vi "Go.vi"() -> ()   [LabVIEW 2011]
uses:
  <vilib>/Math Plots/2D Math Plots/2D Compass/2D Compass Datatype/Public/Plot Helper (Vector).vi
  <vilib>/Utility/file.llb/Read From Spreadsheet File (I64).vi
  <vilib>/Utility/file.llb/Write To Spreadsheet File (I64).vi
  <vilib>/robotics/Navigation/shared/WorldMap/OccupancyGridWorldMap/NI_Robotics_OccupancyGridWorldMap.lvclass
  <vilib>/robotics/Navigation/NI_Robotics_Navigation .lvlib
  <vilib>/robotics/Obstacle Avoidance/Simple Vector Field Histogram/NI_Robotics_Simple Vector Field Histogram.lvlib
  <vilib>/ptbypt/NI_PtbyPt.lvlib
  <vilib>/Math Plots/2D Math Plots/2D Compass/2D Compass Datatype/2D Compass Datatype.lvclass
panel:
  out "currentCoord":cluster{"x curr":i32, "y curr":i32}
  in  "uncertaintyList":u16(ring) caption="uncertainty" items=[" ", "Uncertainty", "Full"]
  in  "startCoord":cluster{"x start":i32, "y start":i32}
  in  "goalCoord":cluster{"x goal":i32, "y goal":i32}
  in  "Stop Button":bool
  in  "dimention":cluster{"x dim":dbl, "y dim":dbl}={"x dim"=100.0, "y dim"=100.0}
  in  "algoritms":u16(ring) items=["", "Dejkstra", "A*"]
  in  "Uncertain":u32(colorbox)=16448250
  in  "path":u32(colorbox) caption="Path"
  in  "goal":u32(colorbox)=16711744 caption="Goal"
  in  "start":u32(colorbox)=3381759 caption="Start"
  in  "invObs":u32(colorbox)=7171459 caption="Invisible"
  in  "visObs":u32(colorbox)=1985280 caption="Visible"
  in  "free":u32(colorbox)=13238105 caption="Free"
  out "enviroment":i32[][](graph)
  out "phArr":dbl[](array[numeric])
  out "magArr":dbl[](array[numeric])
  out "phase":dbl format="%0.2f"
  out "magnitude":dbl format="%0.2f"
  out "uncertainCode":i32
  out "pathCode":i32
  out "invObsCode":i32
  out "goalCode":i32
  out "startCode":i32
  out "visObsCode":i32
  out "freeCode":i32
  in  "?":T1(tab)
  in  "ModeOfGeneration":u16(ring) items=["Auto", "Hand", "Load"]
  in  "Listbox":i32(listbox)=1
  in  "Tree":string[](tree)
  in  "add":bool
  in  "del":bool
  in  "clear":bool
  in  "generation":bool
  in  "Density":i32=5
  in  "save":bool
  out "Scanning":bool=TRUE
  out "ActivePane":bool=TRUE
  in  "Numeric":dbl
  out "RM":bool
  out "LM":bool
  out "Sonar":bool
  out "Gauge":dbl(knob) scale=0.0..1.0
  out "?":dbl
  out "Slide":u8(slide) scale=0.0..100.0
  in  "Scanning Step":dbl=2.0
  out "2D Compass":cluster{dbl[], dbl[]}(graph)
  in  "stop":bool
  in  "Blank Button":bool
  out "path cost":dbl
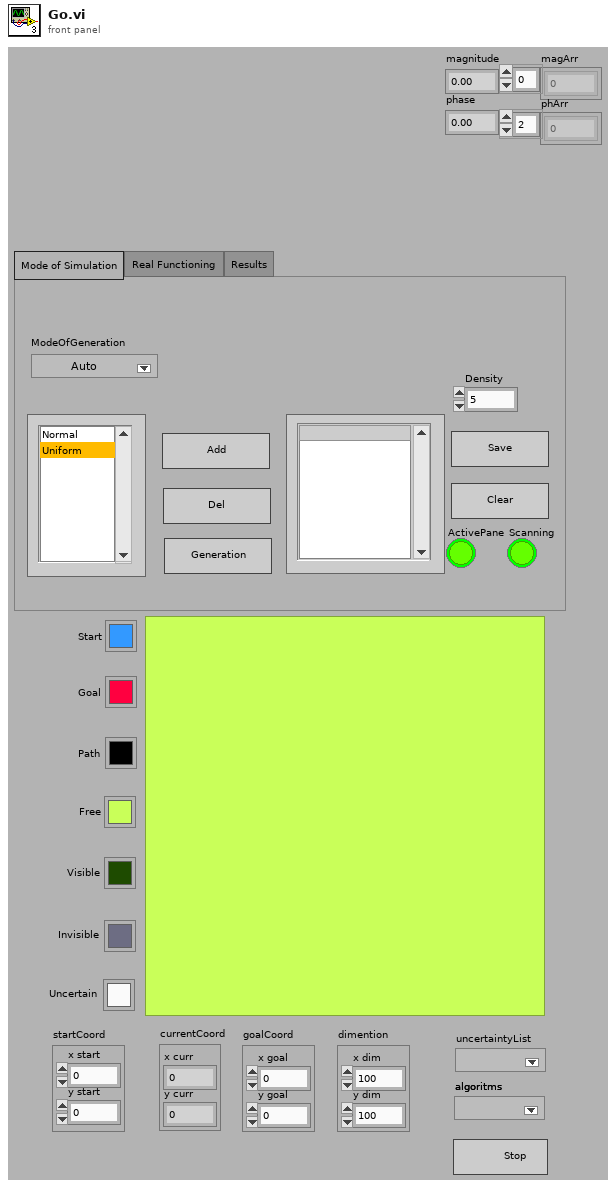
[diagram p1: front panel]
types:
  T1 = enum32{"Mode of Simulation", "Real Functioning ", "Results"}
  T2 = enum8{"Enabled", "Disabled", "Disabled and Grayed Out"}
  T3 = typedef "LVPoint32TypeDef.ctl" = cluster{"Horizontal":i32, "Vertical":i32}
  T4 = cluster{"min mag":dbl, "min phase":dbl, "max phase":dbl, "x relat":i32, "y relat":i32, "visible":bool, "full":bool, "detec":bool}[]
  T5 = typedef "NI_Robotics_Simple Vector Field Histogram.lvlib/Obstacle Description.ctl" = cluster{"angle to obstacle":dbl, "distance to obstacle":dbl}
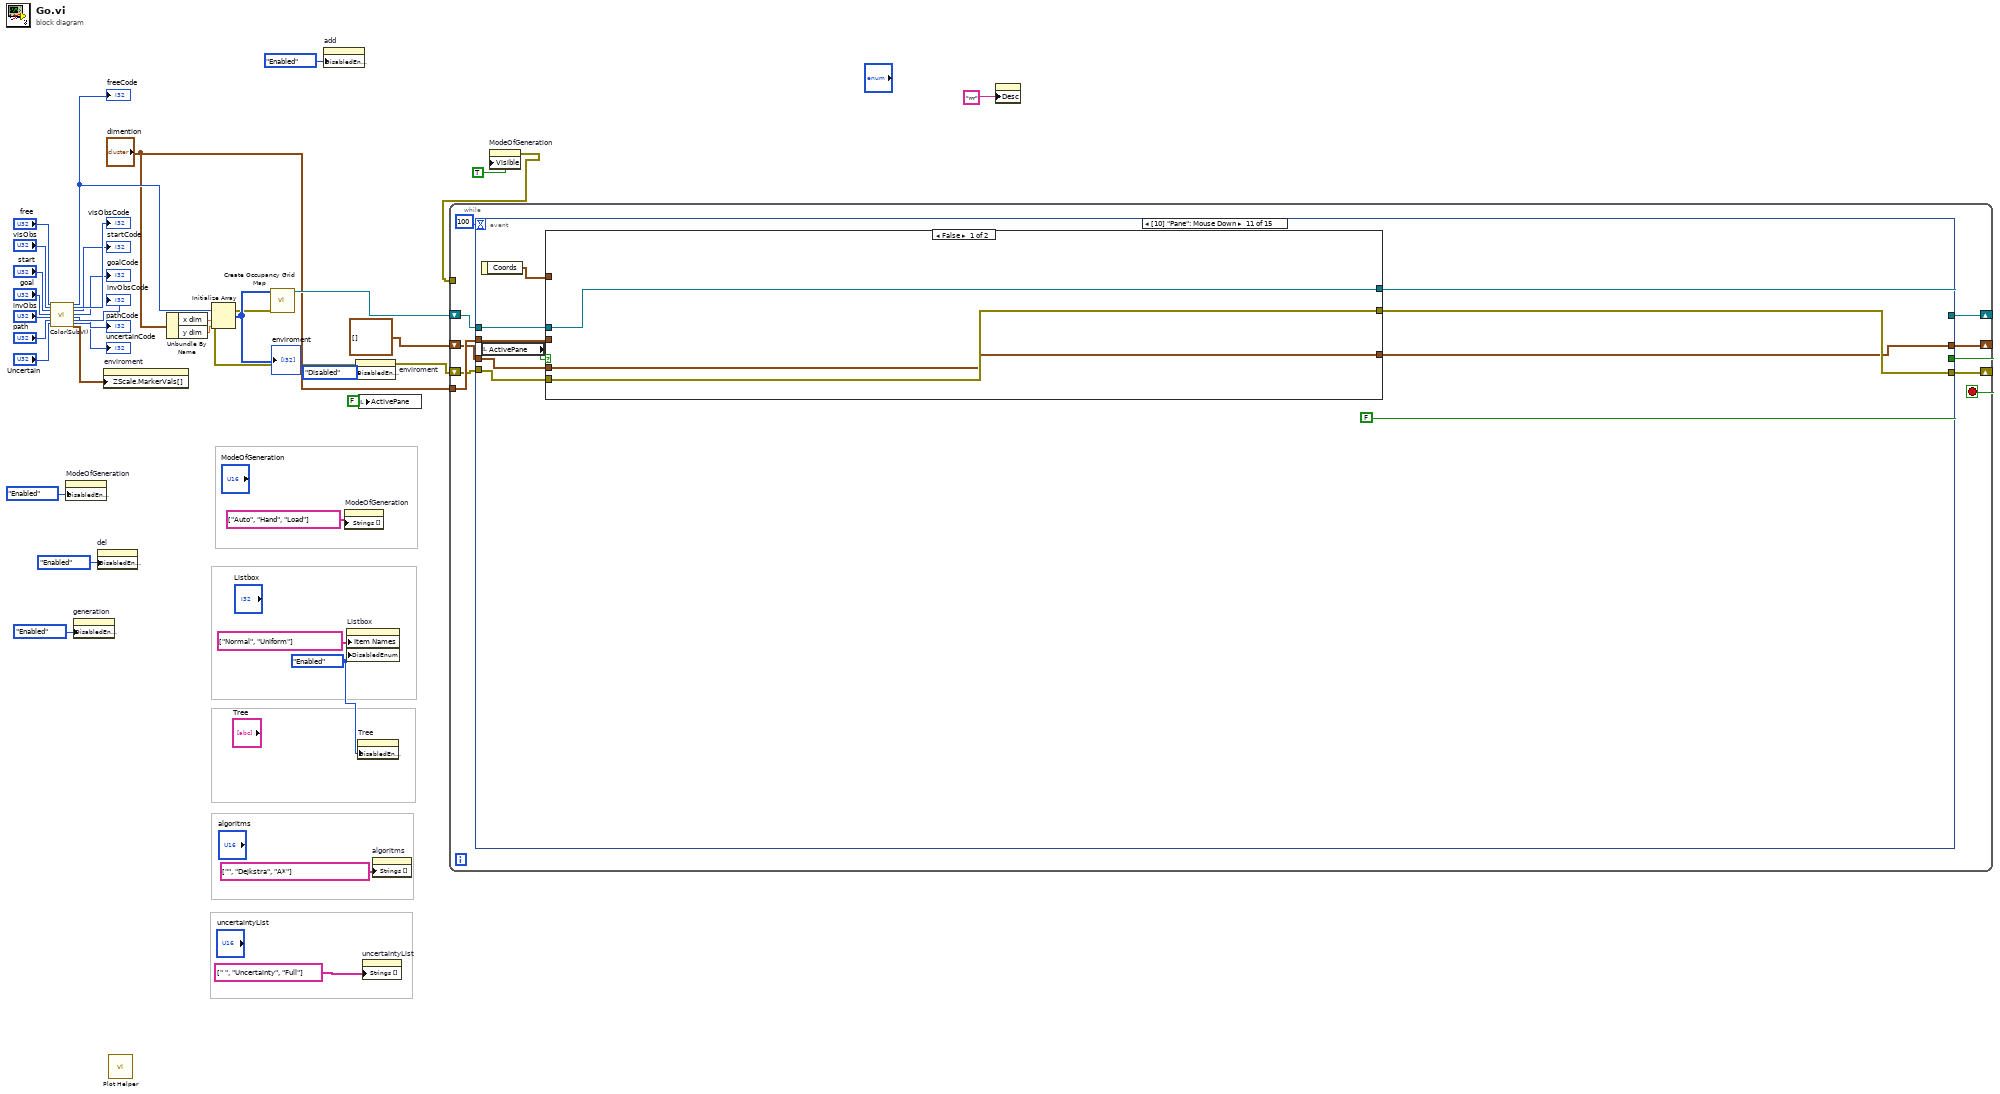
[diagram p0: block diagram]
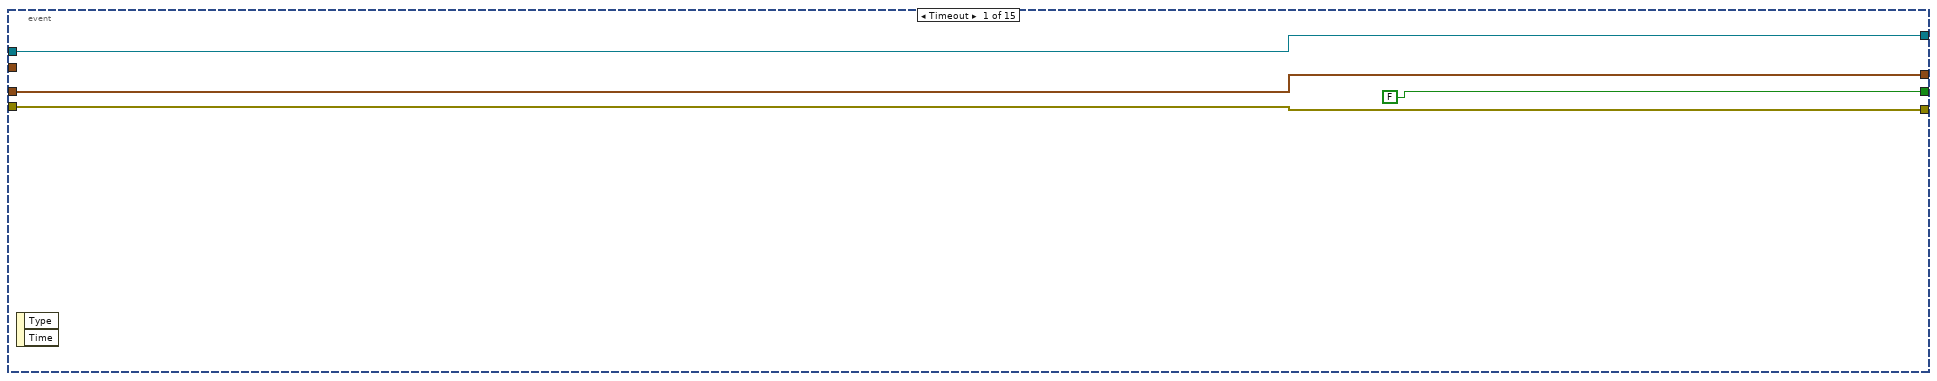
[diagram p2: hidden frame]
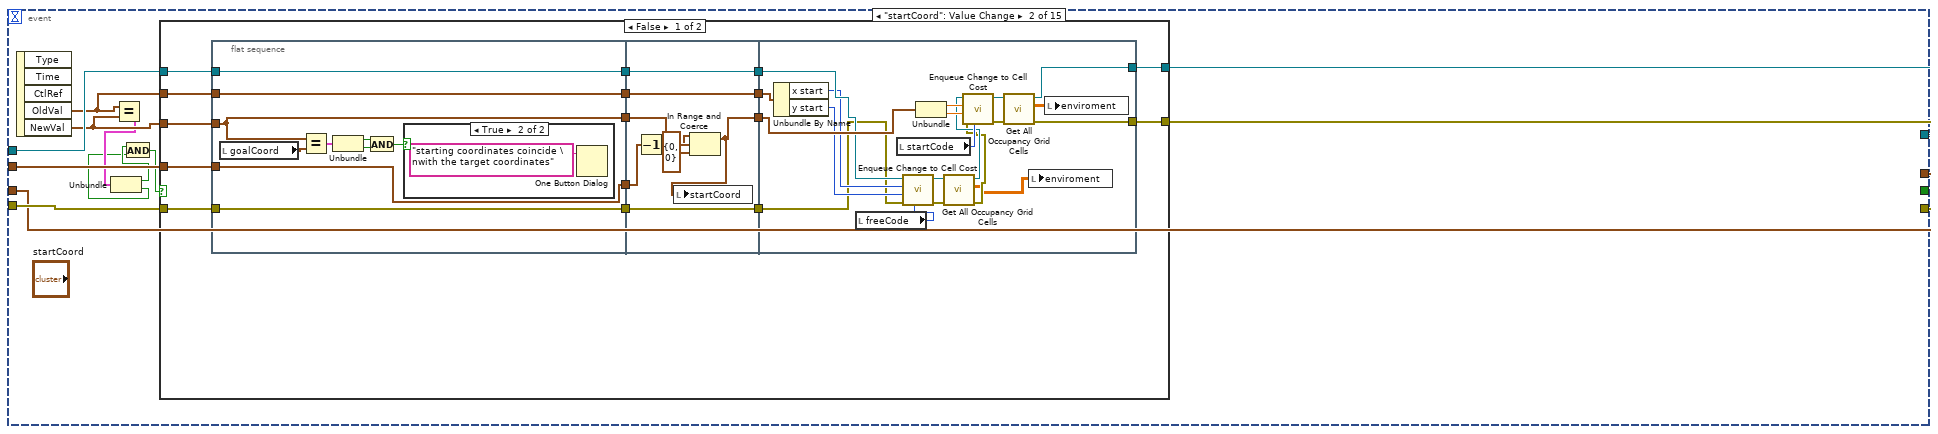
[diagram p3: hidden frame]
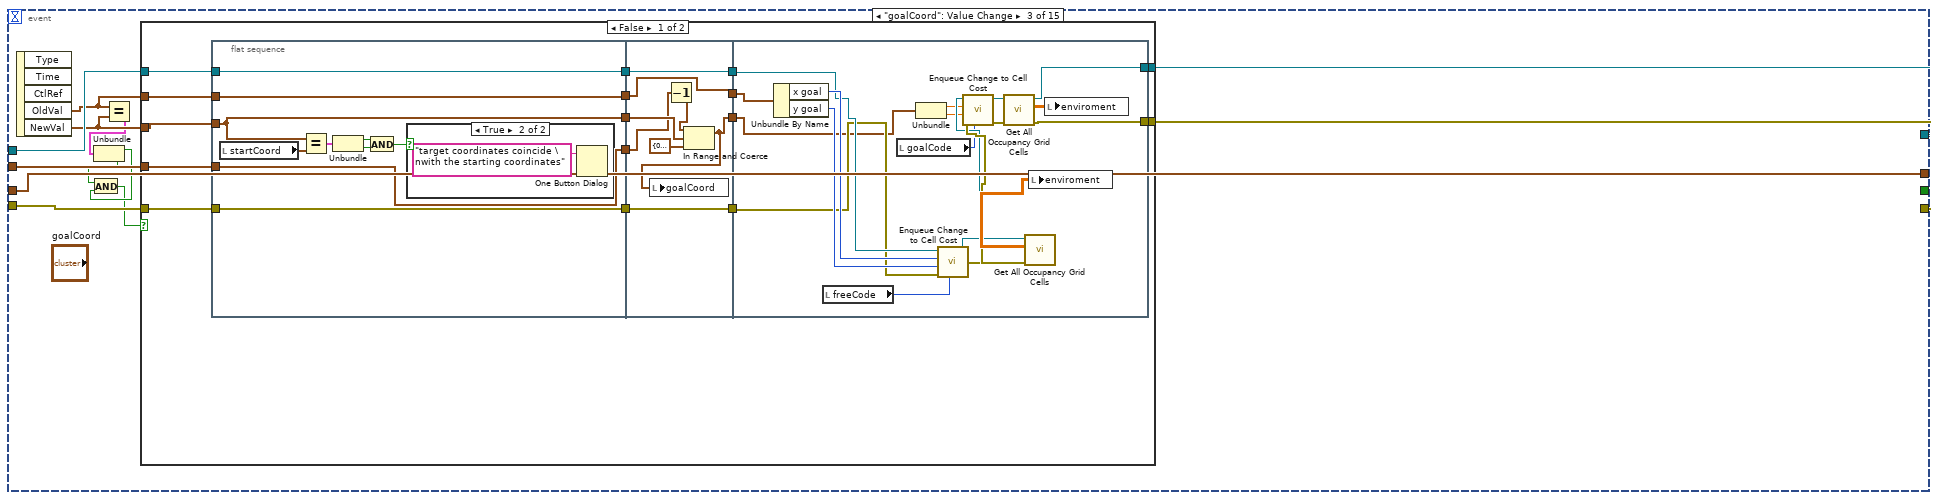
[diagram p6: hidden frame]
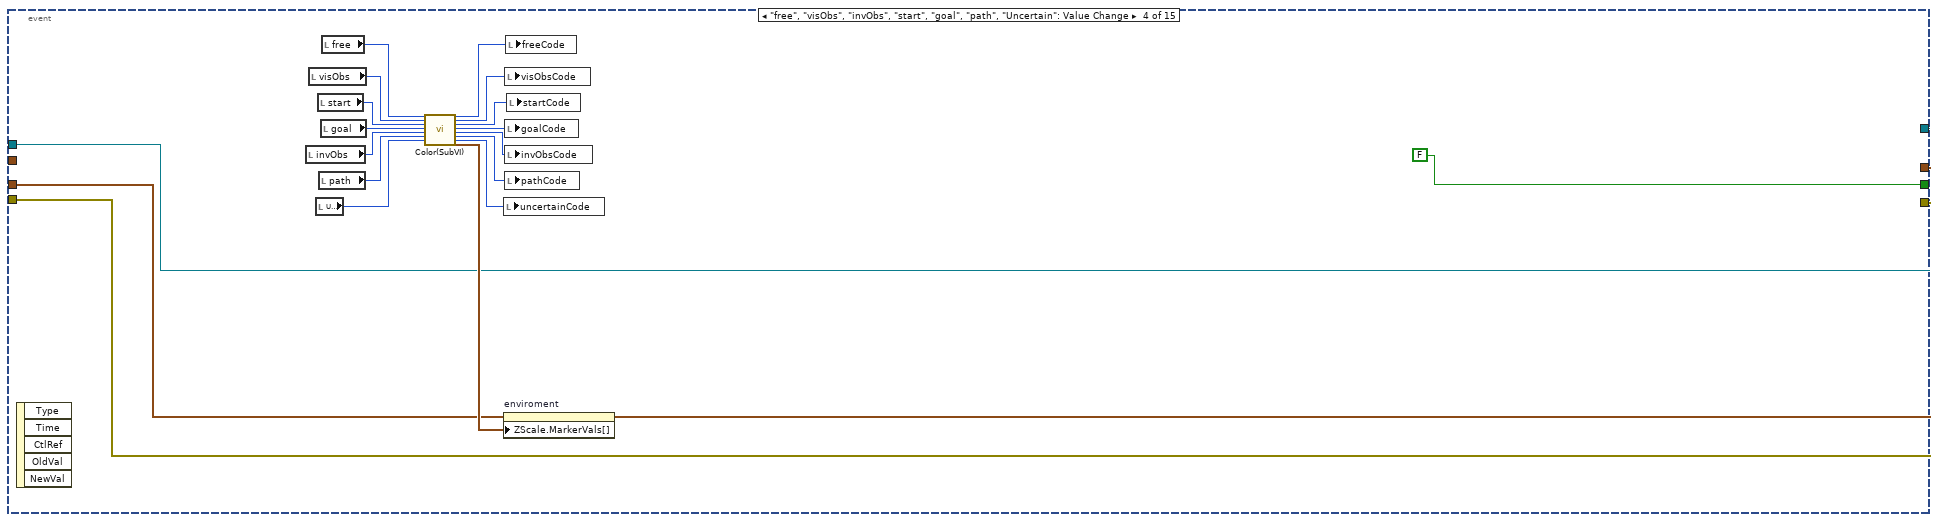
[diagram p9: hidden frame]
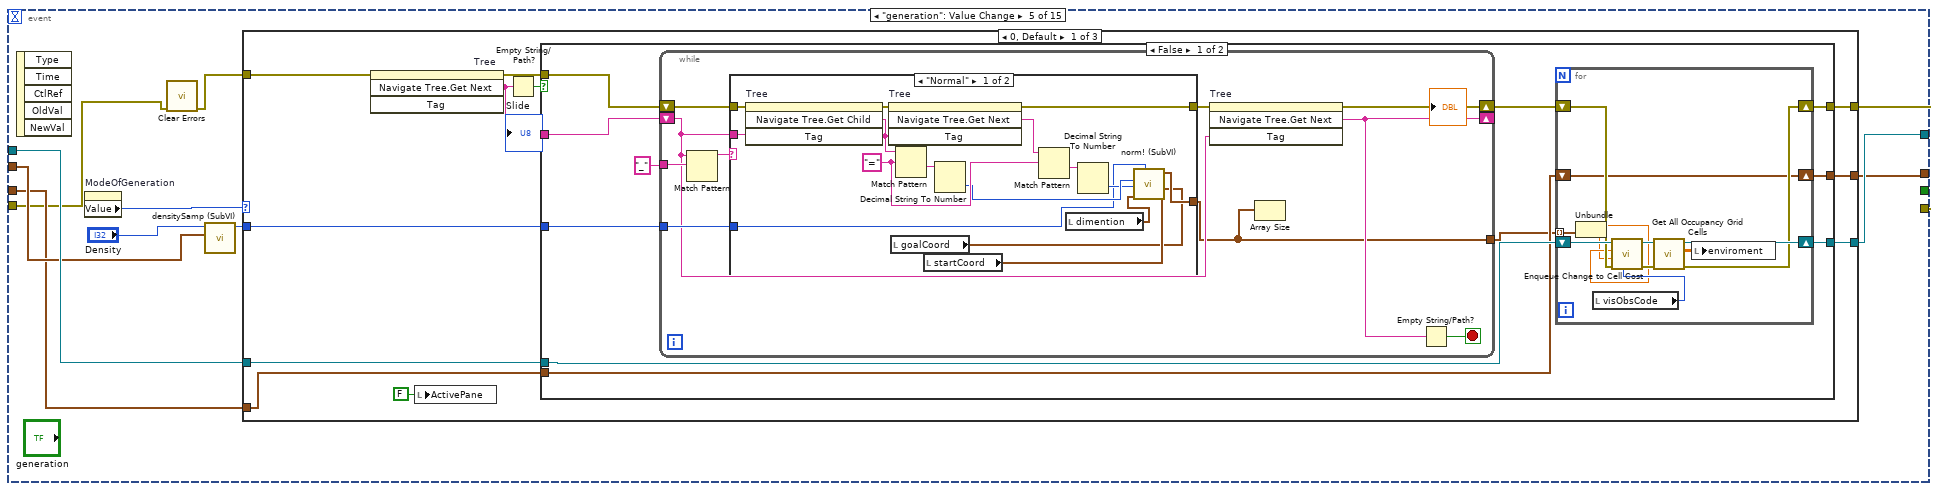
[diagram p10: hidden frame]
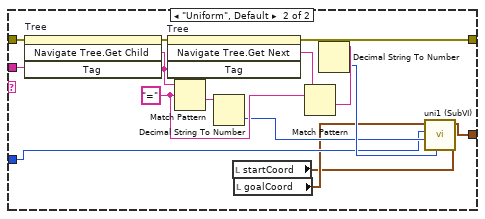
[diagram p11: hidden frame]
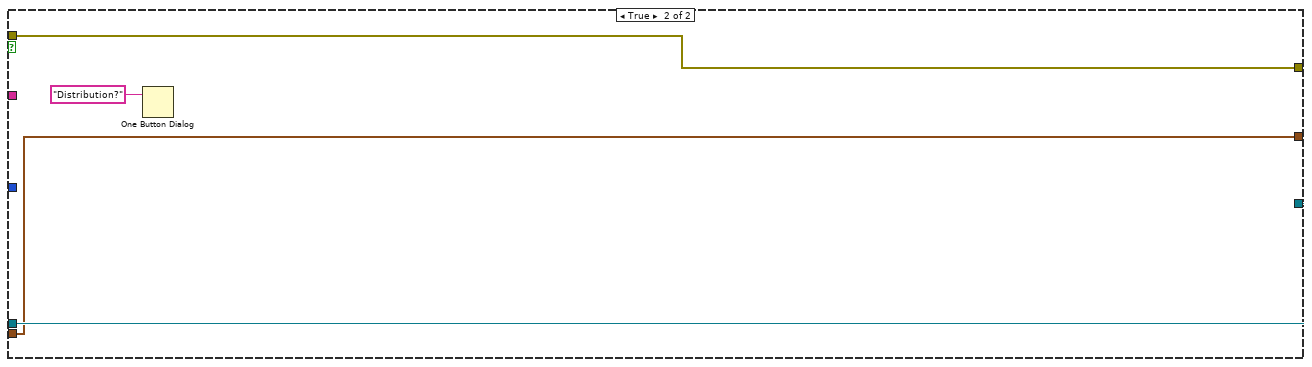
[diagram p12: hidden frame]
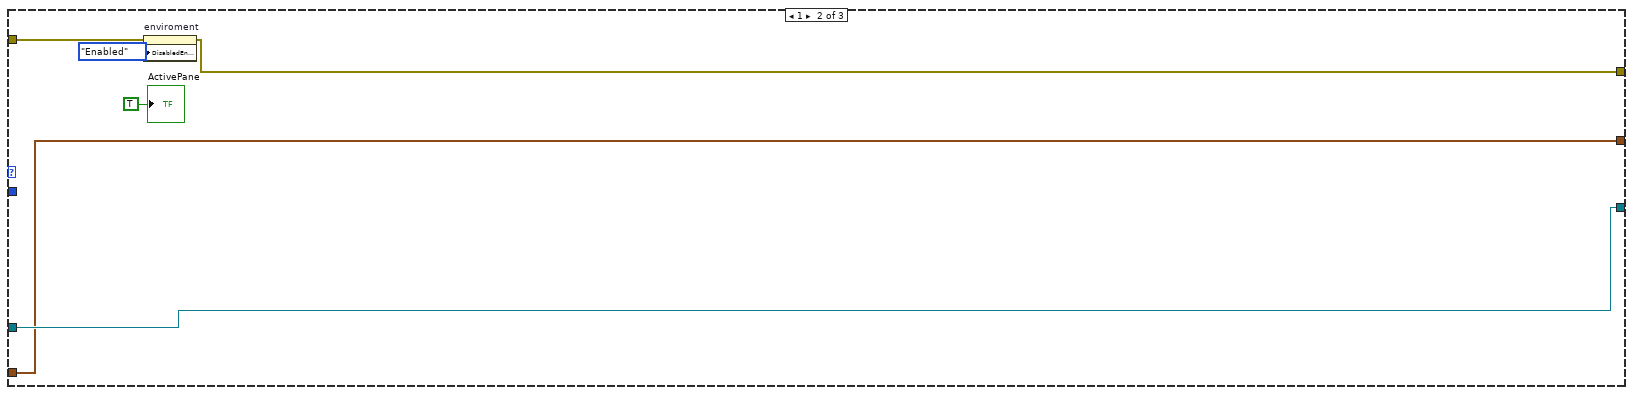
[diagram p13: hidden frame]
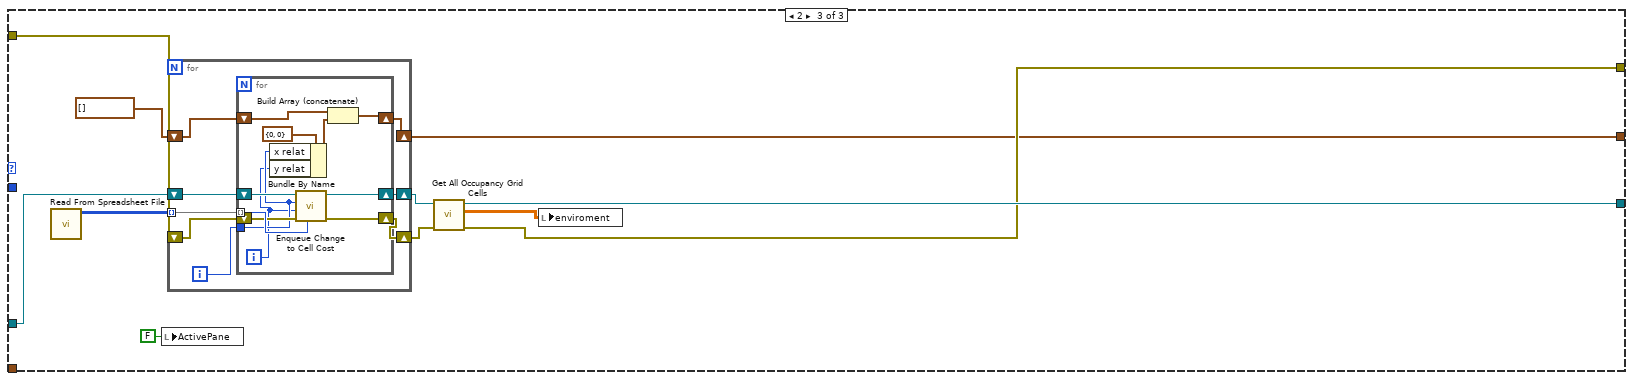
[diagram p14: hidden frame]
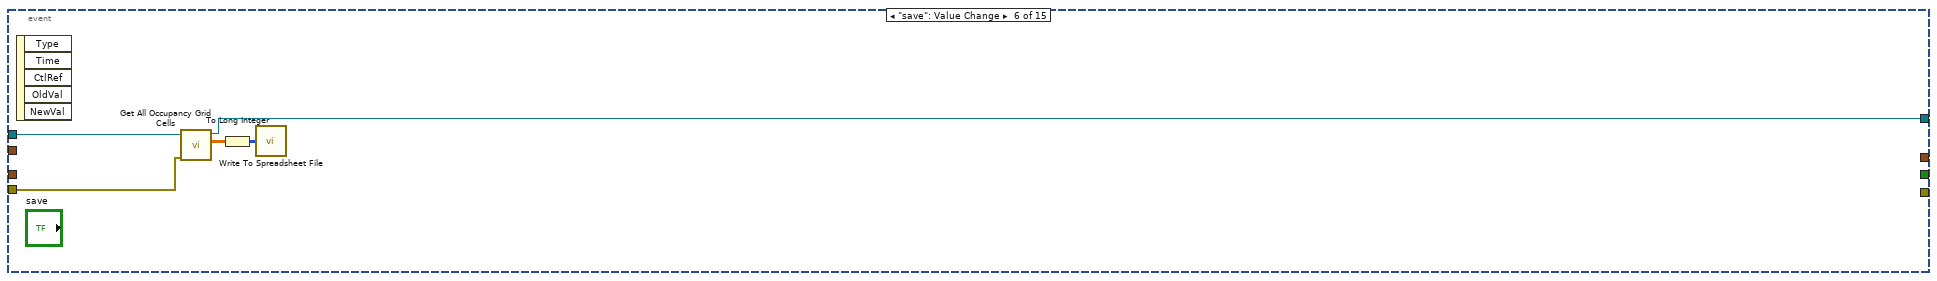
[diagram p15: hidden frame]
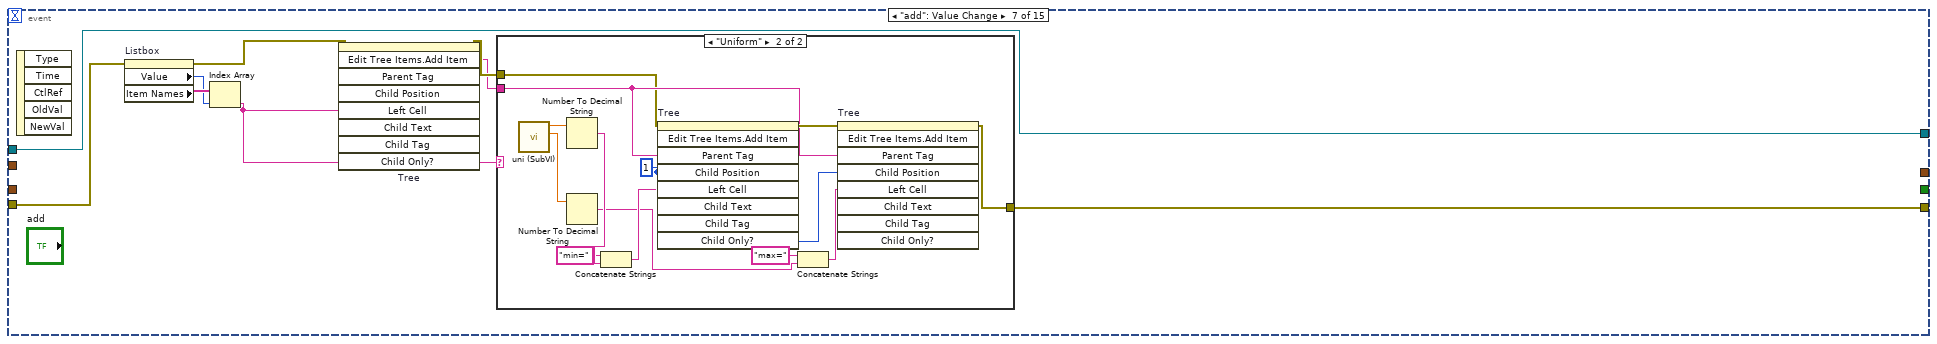
[diagram p16: hidden frame]
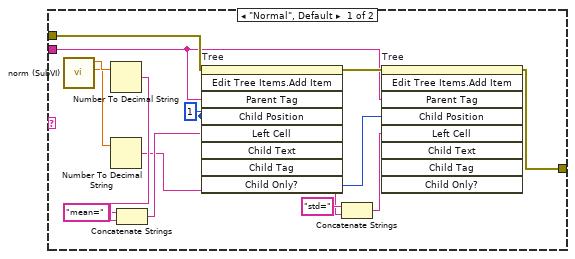
[diagram p17: hidden frame]
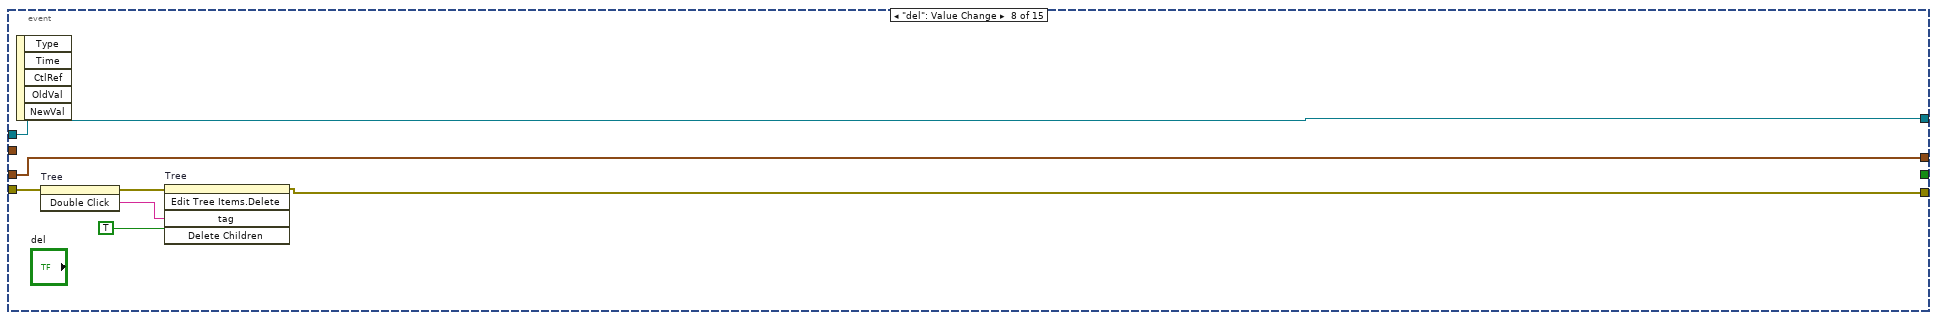
[diagram p18: hidden frame]
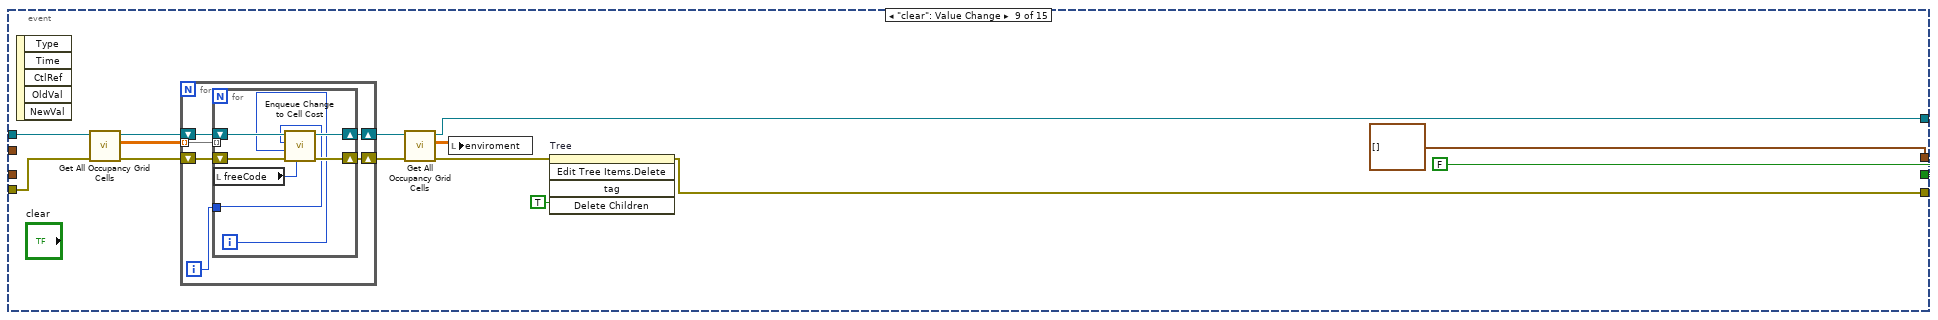
[diagram p19: hidden frame]
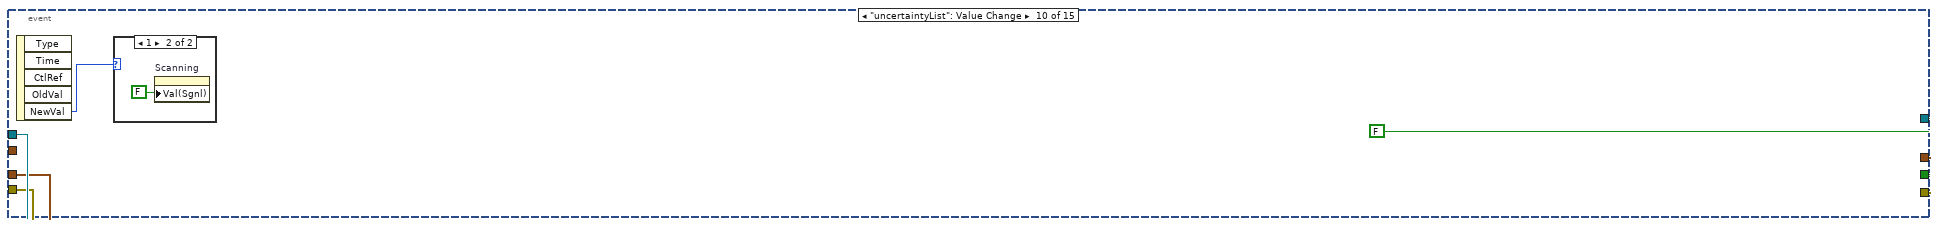
[diagram p20: hidden frame]
diagram:
  w12 = T2."Enabled" ("Disabled")
  n1 = call "Color(SubVI).vi"("free"="free", "visObs"="visObs", "start"="start", "goal"="goal", "invObs"="invObs", "path"="path", "uncertain"="Uncertain") -> ("freeCode"=w21:i32, "visObsCode"=→"visObsCode":i32, "startCode"=→"startCode":i32, "goalCode"=→"goalCode":i32, "invObsCode"=→"invObsCode":i32, "pathCode"=→"pathCode":i32, "uncertainCode"=→"uncertainCode":i32, "ZScale.MarkerVals[]"=w29:cluster{"cost":i32, "color":u32}[])  [unwired: 13 in]
  "freeCode" <- w21
  n2 = property on="ModeOfGeneration" class="Ring (strict)"("DisabledEnum"=T2."Enabled" ("Disabled")) -> ()  [unwired: 2 in, 2 out]
  n3 = property on="generation" class="Bool"("DisabledEnum"=T2."Enabled" ("Disabled")) -> ()  [unwired: 2 in, 2 out]
  n4 = property on="del" class="Bool"("DisabledEnum"=T2."Enabled" ("Disabled")) -> ()  [unwired: 2 in, 2 out]
  n5 = property on="enviroment" class="IntGraph (strict)"("ZScale.MarkerVals[]"=w29) -> ()  [unwired: 2 in, 2 out]
  n6 = call-poly <vilib>:"Plot Helper.vi"() -> ()  [unwired: 4 in, 8 out]
  n7 = Unbundle By Name("dimention") -> ("x dim"=w16:dbl, "y dim"=w15:dbl)
  n8 = Initialize Array(w21, w16, w15) -> (w14:i32[][])
  "enviroment" <- w14
  n9 = call <vilib>:"Create Occupancy Grid Map.vi"("occupancy grid"=w14) -> ("error out"=w10:errorcluster, "map reference out"=w19:refnum<data-value>)  [unwired: 9 in]
  n10 = property on="add" class="Bool"("DisabledEnum"=T2."Enabled" ("Disabled")) -> ()  [unwired: 2 in, 2 out]
  n11 = property on="ModeOfGeneration" class="Ring (strict)"("Strings []"=string[] ["Auto", "Hand", "Load"]) -> ()  [unwired: 2 in, 2 out]
  n12 = property on="Listbox" class="LstBox (strict)"("Item Names"=string[] ["Normal", "Uniform"], "DisabledEnum"=w12) -> ()  [unwired: 2 in, 2 out]
  n13 = property on="enviroment" class="IntGraph (strict)"(error in=w10, "DisabledEnum"=T2."Disabled" ("Disabled")) -> (error out=w9:errorcluster)  [unwired: 1 in, 1 out]
  n14 = property on="Tree" class="Tree (strict)"("DisabledEnum"=w12) -> ()  [unwired: 2 in, 2 out]
  n15 = local write "ActivePane"(FALSE ("Boolean")) -> ()
  n16 = property on="uncertaintyList" class="Ring (strict)"("Strings []"=string[] [" ", "Uncertainty", "Full"]) -> ()  [unwired: 2 in, 2 out]
  n17 = property on="algoritms" class="Ring (strict)"("Strings []"=string[] ["", "Dejkstra", "A*"]) -> ()  [unwired: 2 in, 2 out]
  n18 = property on="ModeOfGeneration" class="Ring (strict)"("Visible"=TRUE) -> (error out=w5:errorcluster)  [unwired: 2 in, 1 out]
  n19 = while {
    tunnel: "dimention" -> [w45]
    shift-right: [w44] -> _
    shift-left: cluster{"x relat ":i32, "y relat":i32}[] [] -> [w43]
    shift-right: [w42] -> _
    shift-left: w19 -> [w40]
    shift-right: [w39] -> _
    shift-left: w9 -> [w41]
    tunnel: w5 -> [_]
    stop <- w46 stop-if-true
    n20 = event shown="[10] \"Pane\": Mouse Down" {
      selector: _ -> [_ _ _ _ _ _ _ _ _ _ _ _ _ _ _]
      dyn-events: _ -> [_ _ _ _ _ _ _ _ _ _ _ _ _ _ _]
      timeout: 100 -> [_ _ _ _ _ _ _ _ _ _ _ _ _ _ _]
      tunnel: w40 -> [w50 w60 w129 w191 w217 w338 w339 w376 w394 w411 w423 w494 w577 _ w645]
      tunnel: [w50 w58 w127 w191 w216 w335 w339 w376 w385 w411 w422 w479 w576 _ w645] -> w42
      tunnel: w41 -> [w48 w62 w131 w190 w209 w337 w344 w377 w393 w409 w416 w493 w572 _ _]
      tunnel: [FALSE _ _ FALSE _ _ _ _ FALSE FALSE FALSE _ _ _ TRUE] -> w46
      tunnel: [w48 w59 w128 w190 w218 _ w340 w374 w390 w409 w421 w474 w575 _ _] -> w39
      tunnel: w45 -> [_ w57 w126 _ w213 _ _ _ _ _ w420 _ _ _ _]
      tunnel: [w47 w61 w130 w189 w210 _ _ w375 cluster{"x relat ":i32, "y relat":i32}[] [] w410 w419 _ w573 _ w644] -> w44
      tunnel: w43 -> [w47 w61 w130 w189 w211 _ _ w375 _ w410 w418 w495 w573 _ w644]
      event Timeout {
        n21 = event-data() -> ()  [unwired: 1 in, 2 out]
      }
      event "startCoord": Value Change {
        n22 = event-data() -> ("OldVal"=w51:cluster{"x start":i32, "y start":i32}, "NewVal"=w56:cluster{"x start":i32, "y start":i32})  [unwired: 1 in, 3 out]
        n23 = Equal?(x=w51, y=w56) -> (x = y?=w55:cluster{"x start":bool, "y start":bool})
        n24 = Unbundle(w55) -> ("x start"=w54:bool, "y start"=w53:bool)
        n25 = And(x=w54, y=w53) -> (x .and. y?=w52:bool)
        n26 = case shown="False" w52 {
          tunnel: w62 -> [w71 w118]
          tunnel: w60 -> [w70 w119]
          tunnel: [w69 w118] -> w59
          tunnel: [w68 w119] -> w58
          tunnel: w56 -> [w67 _]
          tunnel: w57 -> [w66 _]
          tunnel: w51 -> [w65 _]
          frame False {
            n27 = flat-sequence {
              tunnel: [w83] -> w78
              tunnel: [w81] -> w77
              tunnel: [w82] -> w76
              tunnel: w70 -> [w83]
              tunnel: w71 -> [w82]
              tunnel: w67 -> [w81]
              tunnel: w66 -> [w80]
              tunnel: [w80] -> w75
              tunnel: w65 -> [w79]
              tunnel: [w79] -> w64
              tunnel: w78 -> [w97]
              tunnel: [w97] -> w74
              tunnel: w77 -> [w95]
              tunnel: [w93] -> w73
              tunnel: w76 -> [w96]
              tunnel: [w96] -> w72
              tunnel: w75 -> [w92]
              tunnel: w64 -> [w90]
              tunnel: [w90] -> w63
              tunnel: [w109] -> w68
              tunnel: w74 -> [w107]
              tunnel: w73 -> [w110]
              tunnel: [w112] -> w69
              tunnel: w72 -> [w100]
              tunnel: w63 -> [w104]
              frame #0 {
                n28 = local read "goalCoord"() -> (w88:cluster{"x goal":i32, "y goal":i32})
                n29 = Equal?(x=w81, y=w88) -> (x = y?=w87:cluster{bool, bool})
                n30 = Unbundle(w87) -> (w86:bool, w85:bool)
                n31 = And(x=w86, y=w85) -> (x .and. y?=w84:bool)
                n32 = case shown="True" w84 {
                  frame False {
                  }
                  frame True {
                    n33 = One Button Dialog(message="starting coordinates coincide \nwith the target coordinates") -> ()  [unwired: 1 in, 1 out]
                  }
                }
              }
              frame #1 {
                n34 = Decrement(x=w92) -> (x-1=w91:cluster{"x dim":dbl, "y dim":dbl})
                n35 = In Range and Coerce(upper limit=w91, x=w95, lower limit=cluster{"x start":i32, "y start":i32} {"x start"=0, "y start"=0}) -> (coerced(x)=w93:cluster{"x dim":dbl, "y dim":dbl})  [unwired: 1 out]
                n36 = local write "startCoord"(w93) -> ()
              }
              frame #2 {
                n37 = Unbundle By Name(w104) -> ("x start"=w103:i32, "y start"=w102:i32)
                n38 = local read "freeCode"() -> (w101:i32)
                n39 = local read "startCode"() -> (w115:i32)
                n40 = call <vilib>:"Enqueue Change to Cell Cost.vi"("cost"=w101, "error in (no error)"=w100, "y"=w102, "x"=w103, "map reference in"=w107) -> ("error out"=w108:errorcluster, "map reference out"=w105:refnum<data-value>)  [unwired: 5 in]
                n41 = Unbundle(w110) -> ("x dim"=w117:dbl, "y dim"=w116:dbl)
                n42 = call <vilib>:"Get All Occupancy Grid Cells.vi"("error in (no error)"=w108, "map reference in"=w105) -> ("error out"=w99:errorcluster, "occupancy grid"=w98:dbl[][], "map reference out"=w106:refnum<data-value>)  [unwired: 7 in]
                n43 = call <vilib>:"Enqueue Change to Cell Cost.vi"("cost"=w115, "error in (no error)"=w99, "y"=w116, "x"=w117, "map reference in"=w106) -> ("error out"=w114:errorcluster, "map reference out"=w113:refnum<data-value>)  [unwired: 5 in]
                n44 = call <vilib>:"Get All Occupancy Grid Cells.vi"("error in (no error)"=w114, "map reference in"=w113) -> ("error out"=w112:errorcluster, "occupancy grid"=w111:dbl[][], "map reference out"=w109:refnum<data-value>)  [unwired: 7 in]
                n45 = local write "enviroment"(w98) -> ()
                n46 = local write "enviroment"(w111) -> ()
              }
            }
          }
          frame True {
          }
        }
      }
      event "goalCoord": Value Change {
        n47 = event-data() -> ("OldVal"=w120:cluster{"x goal":i32, "y goal":i32}, "NewVal"=w125:cluster{"x goal":i32, "y goal":i32})  [unwired: 1 in, 3 out]
        n48 = Equal?(x=w120, y=w125) -> (x = y?=w124:cluster{"x goal":bool, "y goal":bool})
        n49 = Unbundle(w124) -> ("x goal"=w122:bool, "y goal"=w123:bool)
        n50 = And(x=w123, y=w122) -> (x .and. y?=w121:bool)
        n51 = case shown="False" w121 {
          tunnel: w131 -> [w140 w188]
          tunnel: w129 -> [w139 w187]
          tunnel: [w138 w188] -> w128
          tunnel: [w137 w187] -> w127
          tunnel: w125 -> [w136 _]
          tunnel: w126 -> [w135 _]
          tunnel: w120 -> [w133 _]
          frame False {
            n52 = flat-sequence {
              tunnel: [w152] -> w147
              tunnel: [w150] -> w146
              tunnel: [w151] -> w145
              tunnel: w139 -> [w152]
              tunnel: w140 -> [w151]
              tunnel: w136 -> [w150]
              tunnel: w135 -> [w149]
              tunnel: [w149] -> w144
              tunnel: [w148] -> w134
              tunnel: w133 -> [w148]
              tunnel: w147 -> [w166]
              tunnel: [w166] -> w143
              tunnel: w146 -> [w163]
              tunnel: [w162] -> w142
              tunnel: w145 -> [w165]
              tunnel: [w165] -> w141
              tunnel: w144 -> [w161]
              tunnel: w134 -> [w159]
              tunnel: [w159] -> w132
              tunnel: [w172] -> w137
              tunnel: w143 -> [w170]
              tunnel: w142 -> [w168]
              tunnel: [w173] -> w138
              tunnel: w141 -> [w169]
              tunnel: w132 -> [w171]
              frame #0 {
                n53 = local read "startCoord"() -> (w157:cluster{"x start":i32, "y start":i32})
                n54 = Equal?(x=w150, y=w157) -> (x = y?=w156:cluster{bool, bool})
                n55 = Unbundle(w156) -> (w155:bool, w154:bool)
                n56 = And(x=w155, y=w154) -> (x .and. y?=w153:bool)
                n57 = case shown="True" w153 {
                  frame False {
                  }
                  frame True {
                    n58 = One Button Dialog(message="target coordinates coincide \nwith the starting coordinates") -> ()  [unwired: 1 in, 1 out]
                  }
                }
              }
              frame #1 {
                n59 = Decrement(x=w161) -> (x-1=w160:cluster{"x dim":dbl, "y dim":dbl})
                n60 = In Range and Coerce(upper limit=w160, x=w163, lower limit=cluster{"x dim":dbl, "y dim":dbl} {"x dim"=0.0, "y dim"=0.0}) -> (coerced(x)=w162:cluster{"x dim":dbl, "y dim":dbl})  [unwired: 1 out]
                n61 = local write "goalCoord"(w162) -> ()
              }
              frame #2 {
                n62 = Unbundle By Name(w171) -> ("x goal"=w183:i32, "y goal"=w184:i32)
                n63 = local read "freeCode"() -> (w167:i32)
                n64 = local read "goalCode"() -> (w176:i32)
                n65 = Unbundle(w168) -> ("x dim"=w174:dbl, "y dim"=w175:dbl)
                n66 = call <vilib>:"Enqueue Change to Cell Cost.vi"("cost"=w167, "error in (no error)"=w169, "y"=w184, "x"=w183, "map reference in"=w170) -> ("error out"=w180:errorcluster, "map reference out"=w182:refnum<data-value>)  [unwired: 5 in]
                n67 = call <vilib>:"Get All Occupancy Grid Cells.vi"("error in (no error)"=w180, "map reference in"=w182) -> ("error out"=w185:errorcluster, "occupancy grid"=w186:dbl[][], "map reference out"=w181:refnum<data-value>)  [unwired: 7 in]
                n68 = call <vilib>:"Enqueue Change to Cell Cost.vi"("cost"=w176, "error in (no error)"=w185, "y"=w175, "x"=w174, "map reference in"=w181) -> ("error out"=w177:errorcluster, "map reference out"=w178:refnum<data-value>)  [unwired: 5 in]
                n69 = call <vilib>:"Get All Occupancy Grid Cells.vi"("error in (no error)"=w177, "map reference in"=w178) -> ("error out"=w173:errorcluster, "occupancy grid"=w179:dbl[][], "map reference out"=w172:refnum<data-value>)  [unwired: 7 in]
                n70 = local write "enviroment"(w186) -> ()
                n71 = local write "enviroment"(w179) -> ()
              }
            }
          }
          frame True {
          }
        }
      }
      event "free", "visObs", "invObs", "start", "goal", "path", "Uncertain": Value Change {
        n72 = event-data() -> ()  [unwired: 1 in, 5 out]
        n73 = local read "invObs"() -> (w202:u32)
        n74 = local read "visObs"() -> (w205:u32)
        n75 = local read "Uncertain"() -> (w200:u32)
        n76 = local read "start"() -> (w204:u32)
        n77 = local read "path"() -> (w201:u32)
        n78 = local read "goal"() -> (w203:u32)
        n79 = local read "free"() -> (w206:u32)
        n80 = call "Color(SubVI).vi"("free"=w206, "visObs"=w205, "start"=w204, "goal"=w203, "invObs"=w202, "path"=w201, "uncertain"=w200) -> ("freeCode"=w193:i32, "visObsCode"=w199:i32, "startCode"=w198:i32, "goalCode"=w197:i32, "invObsCode"=w196:i32, "pathCode"=w195:i32, "uncertainCode"=w194:i32, "ZScale.MarkerVals[]"=w192:cluster{"cost":i32, "color":u32}[])  [unwired: 13 in]
        n81 = local write "uncertainCode"(w194) -> ()
        n82 = property on="enviroment" class="IntGraph (strict)"("ZScale.MarkerVals[]"=w192) -> ()  [unwired: 2 in, 2 out]
        n83 = local write "visObsCode"(w199) -> ()
        n84 = local write "goalCode"(w197) -> ()
        n85 = local write "invObsCode"(w196) -> ()
        n86 = local write "pathCode"(w195) -> ()
        n87 = local write "freeCode"(w193) -> ()
        n88 = local write "startCode"(w198) -> ()
      }
      event "generation": Value Change {
        n89 = event-data() -> ()  [unwired: 1 in, 5 out]
        n90 = property on="ModeOfGeneration" class="Ring (strict)"() -> ("Value"=w215:u16)  [unwired: 2 in, 2 out]
        n91 = call <vilib>:"Clear Errors.vi"("error in (no error)"=w209) -> ("error out"=w208:errorcluster)  [unwired: 6 in]
        n92 = call "densitySamp (SubVI).vi"("dimention"=w213, "density"="Density") -> ("samples"=w212:i32)  [unwired: 9 in]
        n93 = case shown="0, Default" w215 {
          tunnel: w208 -> [w222 w302 w311]
          tunnel: [w228 w301 w308] -> w218
          tunnel: w217 -> [w227 w300 w312]
          tunnel: [w226 w300 w309] -> w216
          tunnel: w212 -> [w223 _ _]
          tunnel: w211 -> [w220 w298 _]
          tunnel: [w219 w298 w306] -> w210
          frame 0, Default {
            n94 = invoke on="Tree" class="Tree (strict)" method="Navigate Tree.Get Next"(error in=w222) -> (error out=w229:errorcluster, "Navigate Tree:Get Next Item"=w225:string)  [unwired: 3 in, 2 out]
            n95 = local write "ActivePane"(FALSE ("activePane")) -> ()
            n96 = Empty String/Path?(string/path=w225) -> (empty?=w224:bool)
            n97 = case shown="False" w224 {
              tunnel: w229 -> [w240 w296]
              tunnel: [w237 w296] -> w228
              tunnel: w225 -> [w239 _]
              tunnel: w227 -> [w236 w295]
              tunnel: [w235 w295] -> w226
              tunnel: w223 -> [w233 _]
              tunnel: w220 -> [w232 w294]
              tunnel: [w231 w294] -> w219
              frame False {
                n98 = while {
                  shift-right: [w254] -> _
                  shift-left: w239 -> [w255]
                  shift-right: [w260] -> w238
                  shift-left: w240 -> [w262]
                  tunnel: w233 -> [w258]
                  tunnel: "_" ("string") -> [w257]
                  tunnel: [w253] -> w230
                  stop <- w259 stop-if-true
                  n99 = Match Pattern(string=w255, regular expression=w257) -> (before substring=w256:string)  [unwired: 1 in, 3 out]
                  n100 = case shown="\"Normal\"" w256 {
                    tunnel: w262 -> [w278 w293]
                    tunnel: w255 -> [w276 w291]
                    tunnel: [w275 w290] -> w261
                    tunnel: w258 -> [w265 w281]
                    tunnel: [w269 w284] -> w253
                    frame "Normal" {
                      w272 = "=" ("regular expression")
                      n101 = invoke on="Tree" class="Tree (strict)" method="Navigate Tree.Get Child"(error in=w278, "Tag"=w276) -> (error out=w277:errorcluster, "Navigate Tree:Get Child"=w274:string)  [unwired: 2 in, 2 out]
                      n102 = invoke on="Tree" class="Tree (strict)" method="Navigate Tree.Get Next"(error in=w277, "Tag"=w274) -> (error out=w275:errorcluster, "Navigate Tree:Get Next Item"=w273:string)  [unwired: 2 in, 2 out]
                      n103 = local read "goalCoord"() -> (w263:cluster{"x goal":i32, "y goal":i32})
                      n104 = Match Pattern(string=w274, regular expression=w272) -> (after substring=w271:string)  [unwired: 1 in, 3 out]
                      n105 = local read "startCoord"() -> (w264:cluster{"x start":i32, "y start":i32})
                      n106 = Decimal String To Number(string=w271) -> (number=w268:i32)  [unwired: 2 in, 1 out]
                      n107 = Match Pattern(string=w273, regular expression=w272) -> (after substring=w270:string)  [unwired: 1 in, 3 out]
                      n108 = local read "dimention"() -> (w266:cluster{"x dim":dbl, "y dim":dbl})
                      n109 = Decimal String To Number(string=w270) -> (number=w267:i32)  [unwired: 2 in, 1 out]
                      n110 = call "norm! (SubVI).vi"("start coord"=w264, "goal coord"=w263, "samples"=w265, "upper limit"=w266, "std"=w267, "mean"=w268) -> ("Array"=w269:cluster{"x":dbl, "y":dbl}[])  [unwired: 5 in]
                    }
                    frame "Uniform", Default {
                      w287 = "=" ("regular expression")
                      n111 = invoke on="Tree" class="Tree (strict)" method="Navigate Tree.Get Child"(error in=w293, "Tag"=w291) -> (error out=w292:errorcluster, "Navigate Tree:Get Child"=w289:string)  [unwired: 2 in, 2 out]
                      n112 = invoke on="Tree" class="Tree (strict)" method="Navigate Tree.Get Next"(error in=w292, "Tag"=w289) -> (error out=w290:errorcluster, "Navigate Tree:Get Next Item"=w288:string)  [unwired: 2 in, 2 out]
                      n113 = Match Pattern(string=w289, regular expression=w287) -> (after substring=w286:string)  [unwired: 1 in, 3 out]
                      n114 = Decimal String To Number(string=w286) -> (number=w282:i32)  [unwired: 2 in, 1 out]
                      n115 = local read "startCoord"() -> (w279:cluster{"x start":i32, "y start":i32})
                      n116 = local read "goalCoord"() -> (w280:cluster{"x goal":i32, "y goal":i32})
                      n117 = Match Pattern(string=w288, regular expression=w287) -> (after substring=w285:string)  [unwired: 1 in, 3 out]
                      n118 = Decimal String To Number(string=w285) -> (number=w283:i32)  [unwired: 2 in, 1 out]
                      n119 = call "uni1 (SubVI).vi"("start"=w279, "xmax"=w283, "xmin"=w282, "dencity"=w281, "goal"=w280) -> ("Array"=w284:cluster{"x":dbl, "y":dbl}[])  [unwired: 6 in]
                    }
                  }
                  n120 = invoke on="Tree" class="Tree (strict)" method="Navigate Tree.Get Next"(error in=w261, "Tag"=w255) -> (error out=w260:errorcluster, "Navigate Tree:Get Next Item"=w254:string)  [unwired: 2 in, 2 out]
                  n121 = Array Size(array=w253) -> ()  [unwired: 1 out]
                  n122 = Empty String/Path?(string/path=w254) -> (empty?=w259:bool)
                }
                n123 = for {
                  shift-right: [w249] -> w235
                  shift-left: w236 -> [w248]
                  shift-right: [w246] -> w237
                  shift-left: w238 -> [w247]
                  shift-right: [w241] -> w231
                  shift-left: w232 -> [w241]
                  tunnel: w230 -> [w242] mode=indexing
                  n124 = Unbundle(w242) -> ("x"=w244:dbl, "y"=w243:dbl)
                  n125 = local read "visObsCode"() -> (w252:i32)
                  n126 = call <vilib>:"Enqueue Change to Cell Cost.vi"("cost"=w252, "error in (no error)"=w247, "y"=w243, "x"=w244, "map reference in"=w248) -> ("error out"=w251:errorcluster, "map reference out"=w250:refnum<data-value>)  [unwired: 5 in]
                  n127 = call <vilib>:"Get All Occupancy Grid Cells.vi"("error in (no error)"=w251, "map reference in"=w250) -> ("error out"=w246:errorcluster, "occupancy grid"=w245:dbl[][], "map reference out"=w249:refnum<data-value>)  [unwired: 7 in]
                  n128 = local write "enviroment"(w245) -> ()
                }
              }
              frame True {
                n129 = One Button Dialog(message="Distribution?") -> ()  [unwired: 1 in, 1 out]
              }
            }
          }
          frame 1 {
            n130 = property on="enviroment" class="IntGraph (strict)"(error in=w302, "DisabledEnum"=T2."Enabled" ("Disabled")) -> (error out=w301:errorcluster)  [unwired: 1 in, 1 out]
            "ActivePane" <- TRUE ("Boolean")
          }
          frame 2 {
            n131 = call-poly <vilib>:"Read From Spreadsheet File.vi"() -> ("all rows"=w313:i64[][])  [unwired: 7 in, 4 out]
            n132 = local write "ActivePane"(FALSE ("activePane")) -> ()
            n133 = for {
              tunnel: w313 -> [w322] mode=indexing
              shift-right: [w319] -> w310
              shift-left: w312 -> [w321]
              shift-right: [w318] -> w304
              shift-left: w311 -> [w315]
              shift-right: [w317] -> w306
              shift-left: cluster{"x relat ":i32, "y relat":i32}[] [] -> [w316]
              i -> [w320]
              n134 = for {
                tunnel: w322 -> [w332] mode=indexing
                tunnel: w320 -> [w328]
                shift-right: [w330] -> w319
                shift-left: w321 -> [w333]
                shift-right: [w323] -> w318
                shift-left: w315 -> [w331]
                shift-right: [w325] -> w317
                shift-left: w316 -> [w324]
                i -> [w327]
                n135 = Bundle By Name(cluster=cluster{"x relat ":i32, "y relat":i32} {"x relat "=0, "y relat"=0} ("relatCoord"), "x relat"=w328, "y relat"=w327) -> (w326:cluster{"x relat ":i32, "y relat":i32})
                n136 = call <vilib>:"Enqueue Change to Cell Cost.vi"("cost"=w332, "error in (no error)"=w331, "y"=w327, "x"=w328, "map reference in"=w333) -> ("error out"=w323:errorcluster, "map reference out"=w330:refnum<data-value>)  [unwired: 5 in]
                n137 = Build Array (concatenate)(w324, w326) -> (w325:cluster{"x relat ":i32, "y relat":i32}[])
              }
            }
            n138 = call <vilib>:"Get All Occupancy Grid Cells.vi"("error in (no error)"=w304, "map reference in"=w310) -> ("error out"=w308:errorcluster, "occupancy grid"=w307:dbl[][], "map reference out"=w309:refnum<data-value>)  [unwired: 7 in]
            n139 = local write "enviroment"(w307) -> ()
          }
        }
      }
      event "save": Value Change {
        n140 = event-data() -> ()  [unwired: 1 in, 5 out]
        n141 = call <vilib>:"Get All Occupancy Grid Cells.vi"("error in (no error)"=w337, "map reference in"=w338) -> ("occupancy grid"=w336:dbl[][], "map reference out"=w335:refnum<data-value>)  [unwired: 7 in, 1 out]
        n142 = To Long Integer(number=w336) -> (32bit integer=w334:i32[][])
        n143 = call-poly <vilib>:"Write To Spreadsheet File.vi"("2D data"=w334) -> ()  [unwired: 7 in, 1 out]
      }
      event "add": Value Change {
        n144 = event-data() -> ()  [unwired: 1 in, 5 out]
        n145 = property on="Listbox" class="LstBox (strict)"(error in=w344) -> (error out=w343:errorcluster, "Value"=w346:i32, "Item Names"=w347:string[])  [unwired: 1 in, 1 out]
        n146 = Index Array(array=w347, index=w346) -> (element=w345:string)
        n147 = invoke on="Tree" class="Tree (strict)" method="Edit Tree Items.Add Item"(error in=w343, "Left Cell"=w345) -> (error out=w342:errorcluster, "Edit Tree Items:Add Item"=w341:string)  [unwired: 7 in, 7 out]
        n148 = case shown="\"Uniform\"" w345 {
          tunnel: w342 -> [w360 w363]
          tunnel: w341 -> [w357 w364]
          tunnel: [w348 w361] -> w340
          frame "Normal", Default {
            w356 = 1 ("Child Position")
            n149 = call "norm (SubVI).vi"() -> ("stOut"=w355:dbl, "meanOut"=w359:dbl)  [unwired: 10 in]
            n150 = Number To Decimal String(number=w359) -> (decimal integer string=w354:string)  [unwired: 1 in]
            n151 = Number To Decimal String(number=w355) -> (decimal integer string=w350:string)  [unwired: 1 in]
            n152 = Concatenate Strings("mean=" ("string"), w354) -> (w353:string)
            n153 = invoke on="Tree" class="Tree (strict)" method="Edit Tree Items.Add Item"(error in=w360, "Parent Tag"=w357, "Child Position"=w356, "Left Cell"=w353) -> (error out=w358:errorcluster)  [unwired: 5 in, 8 out]
            n154 = Concatenate Strings("std=" ("string"), w350) -> (w349:string)
            n155 = invoke on="Tree" class="Tree (strict)" method="Edit Tree Items.Add Item"(error in=w358, "Parent Tag"=w357, "Child Position"=w356, "Left Cell"=w349) -> (error out=w348:errorcluster)  [unwired: 5 in, 8 out]
          }
          frame "Uniform" {
            w372 = 1 ("Child Position")
            n156 = call "uni (SubVI).vi"() -> ("maxOut"=w365:dbl, "minOut"=w366:dbl)  [unwired: 8 in]
            n157 = Number To Decimal String(number=w366) -> (decimal integer string=w371:string)  [unwired: 1 in]
            n158 = Number To Decimal String(number=w365) -> (decimal integer string=w362:string)  [unwired: 1 in]
            n159 = Concatenate Strings("min=" ("string"), w371) -> (w370:string)
            n160 = invoke on="Tree" class="Tree (strict)" method="Edit Tree Items.Add Item"(error in=w363, "Parent Tag"=w364, "Child Position"=w372, "Left Cell"=w370) -> (error out=w373:errorcluster)  [unwired: 5 in, 8 out]
            n161 = Concatenate Strings("max=" ("string"), w362) -> (w367:string)
            n162 = invoke on="Tree" class="Tree (strict)" method="Edit Tree Items.Add Item"(error in=w373, "Parent Tag"=w364, "Child Position"=w372, "Left Cell"=w367) -> (error out=w361:errorcluster)  [unwired: 5 in, 8 out]
          }
        }
      }
      event "del": Value Change {
        n163 = event-data() -> ()  [unwired: 1 in, 5 out]
        n164 = invoke on="Tree" class="Tree (strict)" method="Double Click"(error in=w377) -> (error out=w379:errorcluster, "Double Click"=w380:string)  [unwired: 2 in, 1 out]
        n165 = invoke on="Tree" class="Tree (strict)" method="Edit Tree Items.Delete"(error in=w379, "tag"=w380, "Delete Children"=TRUE ("Delete Children?")) -> (error out=w374:errorcluster)  [unwired: 2 in, 4 out]
      }
      event "clear": Value Change {
        n166 = event-data() -> ()  [unwired: 1 in, 5 out]
        n167 = call <vilib>:"Get All Occupancy Grid Cells.vi"("error in (no error)"=w393, "map reference in"=w394) -> ("error out"=w386:errorcluster, "occupancy grid"=w381:dbl[][], "map reference out"=w388:refnum<data-value>)  [unwired: 7 in]
        n168 = for {
          tunnel: w381 -> [w396] mode=indexing
          shift-right: [w399] -> w387
          shift-left: w388 -> [w400]
          shift-right: [w397] -> w384
          shift-left: w386 -> [w398]
          i -> [w395]
          n169 = for {
            tunnel: w396 -> [_] mode=indexing
            tunnel: w395 -> [w402]
            shift-right: [w406] -> w399
            shift-left: w400 -> [w407]
            shift-right: [w404] -> w397
            shift-left: w398 -> [w405]
            i -> [w401]
            n170 = local read "freeCode"() -> (w403:i32)
            n171 = call <vilib>:"Enqueue Change to Cell Cost.vi"("cost"=w403, "error in (no error)"=w405, "y"=w401, "x"=w402, "map reference in"=w407) -> ("error out"=w404:errorcluster, "map reference out"=w406:refnum<data-value>)  [unwired: 5 in]
          }
        }
        n172 = call <vilib>:"Get All Occupancy Grid Cells.vi"("error in (no error)"=w384, "map reference in"=w387) -> ("error out"=w383:errorcluster, "occupancy grid"=w382:dbl[][], "map reference out"=w385:refnum<data-value>)  [unwired: 7 in]
        n173 = local write "enviroment"(w382) -> ()
        n174 = invoke on="Tree" class="Tree (strict)" method="Edit Tree Items.Delete"(error in=w383, "Delete Children"=TRUE ("Delete Children?")) -> (error out=w390:errorcluster)  [unwired: 3 in, 4 out]
      }
      event "uncertaintyList": Value Change {
        n175 = event-data() -> ("NewVal"=w412:u16)  [unwired: 1 in, 4 out]
        n176 = case shown="1" w412 {
          frame 0, Default {
            n177 = property on="Scanning" class="Bool (strict)"("Val(Sgnl)"=TRUE ("scanning")) -> ()  [unwired: 2 in, 2 out]
          }
          frame 1 {
            n178 = property on="Scanning" class="Bool (strict)"("Val(Sgnl)"=FALSE ("scanning")) -> ()  [unwired: 2 in, 2 out]
          }
        }
      }
      event Mouse Down {
        n179 = event-data() -> ("Coords"=w417:T3)  [unwired: 1 in]
        n180 = local read "ActivePane"() -> (w415:bool)
        n181 = case shown="False" w415 {
          tunnel: w423 -> [w427 w452]
          tunnel: [w427 w451] -> w422
          tunnel: [w426 w450] -> w421
          tunnel: w420 -> [_ w449]
          tunnel: [w425 w443] -> w419
          tunnel: w418 -> [w425 w442]
          tunnel: w417 -> [_ w436]
          tunnel: w416 -> [w426 w429]
          frame False {
          }
          frame True {
            w448 = 0.0
            n182 = invoke on="enviroment" class="IntGraph (strict)" method="Map Coords To XY"("Coords"=w436) -> ("XY"=w453:cluster{"X":dbl, "Y":dbl})  [unwired: 6 in, 6 out]
            n183 = Unbundle By Name(w449) -> ("x dim"=w446:dbl, "y dim"=w445:dbl)
            n184 = Decrement(x=w446) -> (x-1=w447:dbl)
            n185 = Decrement(x=w445) -> (x-1=w444:dbl)
            n186 = Round Toward -Infinity(1:w453) -> (0:w437:cluster{"X":dbl, "Y":dbl})
            n187 = local read "goalCoord"() -> (w441:cluster{"x goal":i32, "y goal":i32})
            n188 = local read "startCoord"() -> (w428:cluster{"x start":i32, "y start":i32})
            n189 = Unbundle By Name(w437) -> ("X"=w435:dbl, "Y"=w434:dbl)
            n190 = call "Coinc (SubVI).vi"("paneCoord"=w437, "goalCoord"=w441, "startCoord"=w428) -> ("goalCoinc"=w439:bool, "startCoinc"=w440:bool)  [unwired: 7 in]
            n191 = In Range and Coerce(upper limit=w447, x=w435, lower limit=w448) -> (In Range?=w431:bool)  [unwired: 1 out]
            n192 = In Range and Coerce(upper limit=w444, x=w434, lower limit=w448) -> (In Range?=w430:bool)  [unwired: 1 out]
            n193 = Not(x=w439) -> (.not. x?=w433:bool)
            n194 = Not(x=w440) -> (.not. x?=w432:bool)
            n195 = Compound Arithmetic op=AND(w433, w432, w431, w430) -> (w438:bool)
            n196 = case shown="True" w438 {
              tunnel: w452 -> [w456 w471]
              tunnel: w435 -> [_ w457]
              tunnel: w434 -> [_ w461]
              tunnel: w429 -> [w455 w470]
              tunnel: [w456 w466] -> w451
              tunnel: [w455 w465] -> w450
              tunnel: [w454 w463] -> w443
              tunnel: w442 -> [w454 w462]
              tunnel: w437 -> [_ w460]
              tunnel: w428 -> [_ w459]
              frame False {
              }
              frame True {
                n197 = local read "visObsCode"() -> (w464:i32)
                n198 = call "priorCoord (SubVI).vi"("startCoord"=w459, "paneCoord"=w460) -> ("relatCoord"=w458:cluster{"x relat ":i32, "y relat":i32})  [unwired: 9 in]
                n199 = Build Array (concatenate)(w458, w462) -> (w463:cluster{"x relat ":i32, "y relat":i32}[])
                n200 = call <vilib>:"Enqueue Change to Cell Cost.vi"("cost"=w464, "error in (no error)"=w470, "y"=w461, "x"=w457, "map reference in"=w471) -> ("error out"=w468:errorcluster, "map reference out"=w469:refnum<data-value>)  [unwired: 5 in]
                n201 = call <vilib>:"Get All Occupancy Grid Cells.vi"("error in (no error)"=w468, "map reference in"=w469) -> ("error out"=w465:errorcluster, "occupancy grid"=w467:dbl[][], "map reference out"=w466:refnum<data-value>)  [unwired: 7 in]
                n202 = local write "enviroment"(w467) -> ()
              }
            }
          }
        }
      }
      event "Scanning": Value Change {
        n203 = event-data() -> ()  [unwired: 1 in, 5 out]
        n204 = call "visObs (SubVI).vi"("obsts"=w495) -> ("invisObsts"=w492:T4)
        n205 = for {
          tunnel: w492 -> [w502] mode=indexing
          shift-right: [w508] -> w480
          shift-left: w494 -> [w511]
          shift-right: [w507] -> w478
          shift-left: w493 -> [w506]
          shift-right: [w501] -> _
          shift-left: cluster{"x":i32, "y":i32}[] [] -> [w500]
          tunnel: [w499] -> w486
          tunnel: [w498] -> w485
          n206 = Unbundle By Name(w502) -> ("x relat"=w510:i32, "y relat"=w509:i32, "visible"=w504:bool, "full"=w503:bool)
          n207 = And(x=w504, y=w503) -> (x .and. y?=w505:bool)
          n208 = case shown="False" w505 {
            tunnel: w511 -> [w525 w570]
            tunnel: w510 -> [w521 _]
            tunnel: w509 -> [w520 _]
            tunnel: [w522 w570] -> w508
            tunnel: w506 -> [w524 w569]
            tunnel: [w523 w569] -> w507
            tunnel: w503 -> [w519 _]
            tunnel: w502 -> [_ w568]
            tunnel: [w518 w565] -> w501
            tunnel: w500 -> [w518 w564]
            tunnel: [w514 w561] -> w499
            tunnel: [w515 w560] -> w498
            frame False {
              n209 = local read "phase"() -> (w516:dbl)
              n210 = local read "phArr"() -> (w513:dbl[])
              n211 = case shown="False" w519 {
                tunnel: w525 -> [w539 w554]
                tunnel: w524 -> [w536 w551]
                tunnel: [w535 w550] -> w523
                tunnel: [w534 w549] -> w522
                tunnel: w521 -> [w529 w545]
                tunnel: w520 -> [w528 w544]
                frame False {
                  n212 = local read "invObsCode"() -> (w540:i32)
                  n213 = local read "startCoord"() -> (w532:cluster{"x start":i32, "y start":i32})
                  n214 = Unbundle By Name(w532) -> ("x start"=w527:i32, "y start"=w526:i32)
                  n215 = call <vilib>:"Enqueue Change to Cell Cost.vi"("cost"=w540, "error in (no error)"=w536, "y"=w526, "x"=w527, "map reference in"=w539) -> ("error out"=w537:errorcluster, "map reference out"=w538:refnum<data-value>)  [unwired: 5 in]
                  n216 = call <vilib>:"Get All Occupancy Grid Cells.vi"("error in (no error)"=w537, "map reference in"=w538) -> ("error out"=w535:errorcluster, "occupancy grid"=w533:dbl[][], "map reference out"=w534:refnum<data-value>)  [unwired: 7 in]
                  n217 = local write "enviroment"(w533) -> ()
                  n218 = call <vilib>:"1D Rectangular to Polar PtByPt.vi"("y"=w528, "x"=w529) -> ("phase"=→"phase":dbl, "magnitude"=→"magnitude":dbl)
                }
                frame True {
                  n219 = local read "startCoord"() -> (w547:cluster{"x start":i32, "y start":i32})
                  n220 = local read "uncertainCode"() -> (w555:i32)
                  n221 = Unbundle By Name(w547) -> ("x start"=w546:i32, "y start"=w543:i32)
                  n222 = Add(x=w546, y=w545) -> (x+y=w542:i32)
                  n223 = Add(x=w543, y=w544) -> (x+y=w541:i32)
                  n224 = call <vilib>:"Enqueue Change to Cell Cost.vi"("cost"=w555, "error in (no error)"=w551, "y"=w541, "x"=w542, "map reference in"=w554) -> ("error out"=w552:errorcluster, "map reference out"=w553:refnum<data-value>)  [unwired: 5 in]
                  n225 = call <vilib>:"Get All Occupancy Grid Cells.vi"("error in (no error)"=w552, "map reference in"=w553) -> ("error out"=w550:errorcluster, "occupancy grid"=w548:dbl[][], "map reference out"=w549:refnum<data-value>)  [unwired: 7 in]
                  n226 = local write "enviroment"(w548) -> ()
                }
              }
              n227 = local read "magnitude"() -> (w517:dbl)
              n228 = Build Array (concatenate)(w513, w516) -> (w515:dbl[])
              n229 = local read "magArr"() -> (w512:dbl[])
              n230 = Build Array (concatenate)(w512, w517) -> (w514:dbl[])
            }
            frame True {
              n231 = Unbundle By Name(w568) -> ("x relat"=w557:i32, "y relat"=w556:i32)
              n232 = call <vilib>:"1D Rectangular to Polar PtByPt.vi"("y"=w556, "x"=w557) -> ("phase"=w562:dbl, "magnitude"=w563:dbl)
              n233 = local read "magArr"() -> (w559:dbl[])
              n234 = local read "phArr"() -> (w558:dbl[])
              n235 = Bundle By Name(cluster=cluster{"x":i32, "y":i32} {"x"=0, "y"=0} ("input cluster"), "x"=w557, "y"=w556) -> (w566:cluster{"x":i32, "y":i32})
              n236 = Build Array (concatenate)(w564, w566) -> (w565:cluster{"x":i32, "y":i32}[])
              n237 = Build Array (concatenate)(w559, w563) -> (w561:dbl[])
              "magArr" <- w561
              n238 = Build Array (concatenate)(w558, w562) -> (w560:dbl[])
              "phArr" <- w560
            }
          }
        }
        n239 = call <vilib>:"Simple Vector Field Histogram.vi"("error in (no error)"=w478, "distance threshold"=2.0, "direction angles"=w485, "distances"=w486) -> ("error out"=w483:errorcluster, "nearest obstacle"=w489:T5)  [unwired: 3 in, 3 out]
        n240 = Unbundle By Name(w489) -> ("angle to obstacle"=w488:dbl, "distance to obstacle"=w487:dbl)
        n241 = flat-sequence {
          tunnel: w475 -> [w496]
          tunnel: [w496] -> w474
          frame #0 {
            w497 = dbl[] [] ("magArr")
            n242 = local write "magArr"(w497) -> ()
            n243 = local write "phArr"(w497) -> ()
          }
        }
        n244 = call <vilib>:"1D Polar to Rectangular PtByPt.vi"("phase"=w488, "magnitude"=w487) -> ("y"=w472:dbl, "x"=w473:dbl)
        n245 = local read "goalCode"() -> (w482:i32)
        n246 = Bundle By Name(cluster=cluster{"xlocalG":dbl, "ylocalG":dbl} {"xlocalG"=1.0, "ylocalG"=1.0} ("input cluster"), "xlocalG"=w473, "ylocalG"=w472) -> ()  [unwired: 1 out]
        n247 = call <vilib>:"Enqueue Change to Cell Cost.vi"("cost"=w482, "error in (no error)"=w483, "y"=w472, "x"=w473, "map reference in"=w480) -> ("error out"=w484:errorcluster, "map reference out"=w481:refnum<data-value>)  [unwired: 5 in]
        n248 = call <vilib>:"Get All Occupancy Grid Cells.vi"("error in (no error)"=w484, "map reference in"=w481) -> ("error out"=w475:errorcluster, "occupancy grid"=w477:dbl[][], "map reference out"=w479:refnum<data-value>)  [unwired: 7 in]
        n249 = local write "enviroment"(w477) -> ()
      }
      event "algoritms": Value Change {
        n250 = event-data() -> ()  [unwired: 1 in, 5 out]
        n251 = property on="algoritms" class="Ring (strict)"(error in=w572) -> (error out=w571:errorcluster, "Value"=w574:u16)  [unwired: 1 in, 1 out]
        n252 = case shown="2" w574 {
          tunnel: w577 -> [w579 w620 w629]
          tunnel: w571 -> [w578 w619 w628]
          tunnel: [w579 w586 w629] -> w576
          tunnel: [w578 w584 w628] -> w575
          frame 0, Default {
          }
          frame 2 {
            n253 = local read "startCoord"() -> (w600:cluster{"x start":i32, "y start":i32})
            n254 = local read "goalCoord"() -> (w601:cluster{"x goal":i32, "y goal":i32})
            n255 = Unbundle By Name(w600) -> ("x start"=w610:i32, "y start"=w609:i32)
            n256 = Unbundle By Name(w601) -> ("x goal"=w608:i32, "y goal"=w607:i32)
            n257 = call <vilib>:"Get Cell Reference.vi"("error in (no error)"=w619, "y"=w609, "x"=w610, "map reference in"=w620) -> ("error out"=w618:errorcluster, "cell reference"=w616:refnum<data-value>, "map reference out"=w617:refnum<data-value>)  [unwired: 4 in, 1 out]
            n258 = call <vilib>:"Get Cell Reference.vi"("error in (no error)"=w618, "y"=w607, "x"=w608, "map reference in"=w617) -> ("error out"=w614:errorcluster, "cell reference"=w615:refnum<data-value>, "map reference out"=w611:refnum<data-value>)  [unwired: 4 in, 1 out]
            n259 = call <vilib>:"A Star Plan.vi"("error in (no error)"=w614, "goal reference"=w615, "start reference"=w616, "map reference in"=w611) -> ("error out"=w613:errorcluster, "path references"=w612:refnum<data-value>[], "path cost"=→"path cost":dbl)  [unwired: 4 in, 1 out]
            n260 = call <vilib>:"Get Cells in Path.vi"("error in (no error)"=w613, "path references"=w612, "map reference in"=w611) -> ("error out"=w603:errorcluster, "y coordinates"=w605:i32[], "x coordinates"=w606:i32[], "map reference out"=w604:refnum<data-value>)  [unwired: 5 in]
            n261 = local read "startCoord"() -> (w595:cluster{"x start":i32, "y start":i32})
            n262 = for {
              tunnel: w606 -> [w626] mode=indexing
              tunnel: w605 -> [w625] mode=indexing
              shift-right: [w622] -> w602
              shift-left: w604 -> [w627]
              shift-right: [w621] -> w591
              shift-left: w603 -> [w624]
              n263 = local read "pathCode"() -> (w623:i32)
              n264 = call <vilib>:"Enqueue Change to Cell Cost.vi"("cost"=w623, "error in (no error)"=w624, "y"=w625, "x"=w626, "map reference in"=w627) -> ("error out"=w621:errorcluster, "map reference out"=w622:refnum<data-value>)  [unwired: 5 in]
            }
            n265 = Unbundle By Name(w595) -> ("x start"=w594:i32, "y start"=w593:i32)
            n266 = local read "goalCoord"() -> (w582:cluster{"x goal":i32, "y goal":i32})
            n267 = local read "startCode"() -> (w592:i32)
            n268 = Unbundle By Name(w582) -> ("x goal"=w581:i32, "y goal"=w580:i32)
            n269 = call <vilib>:"Get All Occupancy Grid Cells.vi"("error in (no error)"=w591, "map reference in"=w602) -> ("map reference out"=w598:refnum<data-value>)  [unwired: 7 in, 2 out]
            n270 = call <vilib>:"Enqueue Change to Cell Cost.vi"("cost"=w592, "error in (no error)"=w591, "y"=w593, "x"=w594, "map reference in"=w598) -> ("error out"=w596:errorcluster, "map reference out"=w597:refnum<data-value>)  [unwired: 5 in]
            n271 = call <vilib>:"Get All Occupancy Grid Cells.vi"("error in (no error)"=w596, "map reference in"=w597) -> ("error out"=w587:errorcluster, "map reference out"=w588:refnum<data-value>)  [unwired: 7 in, 1 out]
            n272 = local read "goalCode"() -> (w583:i32)
            n273 = call <vilib>:"Enqueue Change to Cell Cost.vi"("cost"=w583, "error in (no error)"=w587, "y"=w580, "x"=w581, "map reference in"=w588) -> ("error out"=w589:errorcluster, "map reference out"=w590:refnum<data-value>)  [unwired: 5 in]
            n274 = call <vilib>:"Get All Occupancy Grid Cells.vi"("error in (no error)"=w589, "map reference in"=w590) -> ("error out"=w584:errorcluster, "occupancy grid"=w585:dbl[][], "map reference out"=w586:refnum<data-value>)  [unwired: 7 in]
            n275 = local write "enviroment"(w585) -> ()
          }
          frame 1 {
          }
        }
      }
      event "Blank Button": Value Change {
        n276 = event-data() -> ()  [unwired: 1 in, 5 out]
        n277 = call "111 (SubVI).vi"("scan angle"="Numeric", "step angle"="Scanning Step", "stop"="stop") -> ("sensor"=→"Sonar":bool, "x"=w637:dbl, "Data Value Reference out"=w631:refnum<data-value>, "left motor"=→"LM":bool, "y"=w636:dbl, "right motor"=→"RM":bool, "velocity"=→"Gauge":dbl, "sensor data"=→"2D Compass":cluster{dbl[], dbl[]})  [unwired: 4 in, 1 out]
        n278 = Bundle("x"=w637, "y"=w636) -> (→"currentCoord":cluster{"x":dbl, "y":dbl})  [unwired: 1 in]
        n279 = call <vilib>:"Get All Occupancy Grid Cells.vi"("map reference in"=w631) -> ("occupancy grid"=w632:dbl[][])  [unwired: 8 in, 2 out]
        n280 = local write "enviroment"(w632) -> ()
      }
      event "Stop Button": Value Change {
        n281 = event-data() -> ()  [unwired: 1 in, 5 out]
      }
    }
  }
  n282 = property class="TabCtl (strict)"("Desc"="rrr" ("Description")) -> ()  [unwired: 2 in, 2 out]
